vi "1WIRE_Write_0_bit.vi"(8 "error in":errorcluster) -> (0 "error out":errorcluster)   [LabVIEW 2013]
doc: "This VI is created by Vincent Claes for FPDA-1 more information on http://pwo.fpga.be\n\nvincent.claes@xios.be\nclaesvincent@gmail.com\n\nhttp://www.linkedin.com/in/vincentclaes"
uses:
  <vilib>/eio/EIONode/EIONode.xnode
  <vilib>/eio/EIOMethodNode/EIOMethodNode.xnode
  <vilib>/rvi/eio/common/nirviEmuTemplateMethod_errors.vi
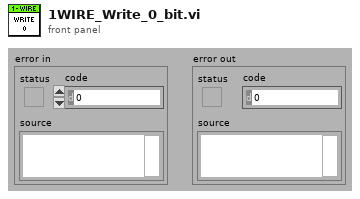
[diagram p1: front panel]
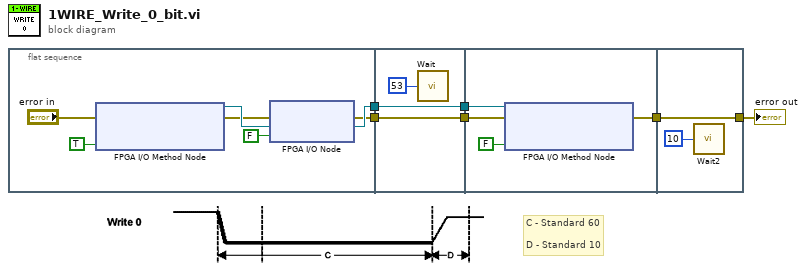
[diagram p0: block diagram]
diagram:
  # "C - Standard 60\n\nD - Standard 10"
  n1 = flat-sequence {
    tunnel: [w11] -> w6
    tunnel: [w8] -> w3
    tunnel: w6 -> [w15]
    tunnel: [w15] -> w5
    tunnel: [w14] -> w4
    tunnel: w3 -> [w14]
    tunnel: w5 -> [w19]
    tunnel: w4 -> [w18]
    tunnel: [w20] -> w2
    tunnel: [w21] -> w1
    tunnel: w2 -> [w21]
    frame #0 {
      n2 = xnode "FPGA I/O Method Node"("error in"="error in", "Enable"=TRUE) -> ("error out"=w9:errorcluster, "FPGA I/O Out"=w12:refnum<k21>)  [unwired: 1 in]
      n3 = xnode "FPGA I/O Node"("error in"=w9, "I/O Item"=FALSE ("FX2_IO1_J1_0"), "FPGA I/O In"=w12) -> ("error out"=w8:errorcluster, "FPGA I/O Out"=w11:refnum<k21>)
    }
    frame #1 {
      n4 = call "Wait"("Count(uSec)"=u32 53) -> ()  [unwired: 1 out]
    }
    frame #2 {
      n5 = xnode "FPGA I/O Method Node"("error in"=w18, "FPGA I/O In"=w19, "Enable"=FALSE) -> ("error out"=w20:errorcluster)  [unwired: 1 out]
    }
    frame #3 {
      n6 = call "Wait2"("Count(uSec)"=u32 10) -> ()  [unwired: 1 out]
    }
  }
  "error out" <- w1
